vi "Test Copy All Funnels.vi"(8 "error in (no error)":errorcluster) -> (0 "error out":errorcluster)   [LabVIEW 2019]
uses:
  Setting Database/Setting Database.lvclass
  C:/Program Files (x86)/National Instruments/LabVIEW 2019/vi.lib/JKI/JKI SMO/SMO/SMO.lvclass
  Setting Database/Typedefs/PrivateEvents--Setting Database.CopyActiveFunnelToAll.ctl
  ObjectSettings/ObjectSettings.lvclass/ObjectSettings.ctl
  ObjectSettings/Accessors/Read Enabled.vi
  ObjectSettings/Accessors/Write Enabled.vi
  Funnel Settings/Funnel Settings.lvclass
  C:/Users/Albro/Documents/GitHub/AFM-Lithography/lvsrc/Classes/Settings/ObjectSettings/ObjectSettings.lvclass
  <vilib>/addons/_JKI Toolkits/Caraya/classes/Assert/Assert Equal Value_Variant.vi
  <vilib>/addons/_JKI Toolkits/Caraya/classes/Assert/Assert Not Error.vi
  <vilib>/addons/_JKI Toolkits/Caraya/classes/Test/Test.lvclass
  <vilib>/addons/_JKI Toolkits/Caraya/classes/Assert/Assert.lvclass
  <vilib>/JKI/JKI SMO/SMO/SMO.lvclass
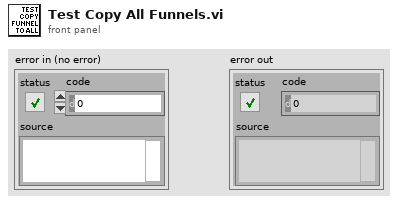
[diagram p1: front panel]
types:
  T1 = typedef "Setting Database.lvclass/PrivateEvents--Setting Database.CopyActiveFunnelToAll.ctl" = bool
  T2 = typedef "Setting Database.lvclass/PublicEvents--Cluster.ctl" = cluster{"NewActivePath":refnum<user-event>, "PathsUpdated":refnum<user-event>, "RectanglesUpdated":refnum<user-event>, "NewActiveRectangle":refnum<user-event>, "NewActiveFunnel":refnum<user-event>, "FunnelsUpdated":refnum<user-event>, "NewActiveDot":refnum<user-event>, "DotsUpdated":refnum<user-event>}
  T3 = typedef "Setting Database.lvclass/PrivateEvents--Setting Database.Refresh.ctl" = cluster{"Paths":string[], "Rectangles":string[], "Funnels":string[], "Dots":string[]}
  T4 = typedef "Setting Database.lvclass/PublicEvents--Setting Database.NewActiveFunnel.ctl" = refnum<class "Funnel Settings.lvclass">
  T5 = typedef "Setting Database.lvclass/PublicEvents--Setting Database.FunnelsUpdated.ctl" = refnum<class "Funnel Settings.lvclass">[]
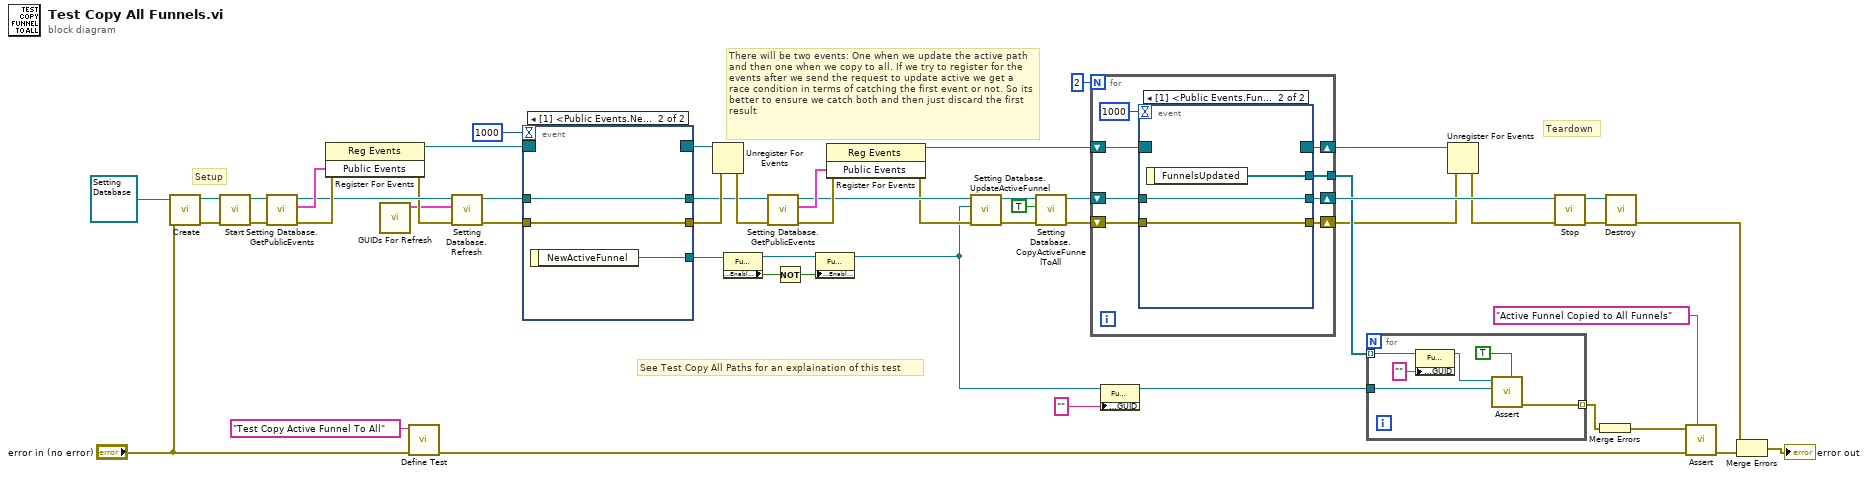
[diagram p0: block diagram]
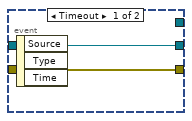
[diagram p2: hidden frame]
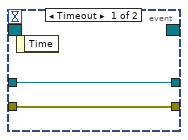
[diagram p3: hidden frame]
diagram:
  # "See Test Copy All Paths for an explaination of this test"
  # "There will be two events: One when we update the active path and then one when we copy to all. If we try to register for the events after we send the request to update active we get a race condition in terms of catching the first event or not. So its better to ensure we catch both and then just discard the first result"
  # "Teardown"
  # "Setup"
  n1 = call <vilib>:"Create.vi"("error in (no error)"="error in (no error)", "SMO"=refnum<class "Setting Database.lvclass"> refnum ("Setting Database.lvclass")) -> ("error out"=w49:errorcluster, "SMO out"=w40:refnum<class "Setting Database.lvclass">)  [unwired: 7 in, 1 out]
  n2 = call <vilib>:"Start.vi"("error in (no error)"=w49, "SMO"=w40) -> ("error out"=w48:errorcluster, "SMO out"=w39:refnum<class "Setting Database.lvclass">)  [unwired: 8 in]
  n3 = call "Setting Database.GetPublicEvents.vi"("error in (no error)"=w48, "Setting Database"=w39) -> ("error out"=w45:errorcluster, "Public Events"=w34:T2, "Setting Database out"=w32:refnum<class "Setting Database.lvclass">)  [unwired: 7 in]
  n4 = register-events(error in=w45, w34) -> (reference out=w35:refnum<event-registration>, error out=w31:errorcluster)  [unwired: 1 in]
  n5 = call "GUIDs For Refresh.vi"() -> ("Initialize"=w4:T3)  [unwired: 10 in, 1 out]
  n6 = call <vilib>:"Define Test.vi"("error in (no error)"="error in (no error)", "Label (VI Title)"="Test Copy Active Funnel To All") -> ("error out"=w51:errorcluster)  [unwired: 8 in, 1 out]
  n7 = call "Setting Database.Refresh.vi"("error in (no error)"=w31, "Initialize"=w4, "Setting Database"=w32) -> ("error out"=w30:errorcluster, "Setting Database out"=w29:refnum<class "Setting Database.lvclass">)  [unwired: 7 in]
  n8 = event shown="[1] <Public Events.NewActiveFunnel>: User Event" {
    selector: w35 -> [_ _]
    dyn-events: [_ _] -> w37
    timeout: 1000 -> [_ _]
    tunnel: [w54 w57] -> w46
    tunnel: w30 -> [w54 w57]
    tunnel: w29 -> [w53 w56]
    tunnel: [w53 w56] -> w17
    tunnel: [_ w55] -> w28
    event Timeout {
      n9 = event-data() -> ()  [unwired: 1 in, 1 out]
    }
    event User Event {
      n10 = event-data() -> ("NewActiveFunnel"=w55:T4)  [unwired: 1 in]
    }
  }
  n11 = Unregister For Events(event registration refnum=w37, error in=w46) -> (error out=w18:errorcluster)
  n12 = property on="Property Node" class="Funnel Settings.lvclass"(reference=w28) -> (reference out=w27:T4, "Accessors:Enabled"=w26:bool)  [unwired: 1 in, 1 out]
  n13 = call "Setting Database.GetPublicEvents.vi"("error in (no error)"=w18, "Setting Database"=w17) -> ("error out"=w16:errorcluster, "Public Events"=w24:T2, "Setting Database out"=w11:refnum<class "Setting Database.lvclass">)  [unwired: 7 in]
  n14 = Not(x=w26) -> (.not. x?=w25:bool)
  n15 = property on="Property Node" class="Funnel Settings.lvclass"(reference=w27, "Accessors:Enabled"=w25) -> (reference out=w2:T4)  [unwired: 1 in, 1 out]
  n16 = register-events(error in=w16, w24) -> (reference out=w22:refnum<event-registration>, error out=w10:errorcluster)  [unwired: 1 in]
  n17 = call "Setting Database.UpdateActiveFunnel.vi"("error in (no error)"=w10, "UpdateActiveFunnel"=w2, "Setting Database"=w11) -> ("error out"=w7:errorcluster, "Setting Database"=w9:refnum<class "Setting Database.lvclass">)  [unwired: 7 in]
  n18 = call "Setting Database.CopyActiveFunnelToAll.vi"("error in (no error)"=w7, "CopyActiveFunnelToAll"=T1 TRUE, "Setting Database"=w9) -> ("error out"=w6:errorcluster, "Setting Database out"=w8:refnum<class "Setting Database.lvclass">)  [unwired: 7 in]
  n19 = for {
    N: 2 -> [_]
    tunnel: [w60] -> w21
    shift-right: [w64] -> w23
    shift-left: w8 -> [w65]
    shift-right: [w63] -> w13
    shift-left: w6 -> [w62]
    shift-right: [w59] -> w14
    shift-left: w22 -> [w61]
    n20 = event shown="[1] <Public Events.FunnelsUpdated>: User Event" {
      selector: w61 -> [_ _]
      dyn-events: [_ _] -> w59
      timeout: 1000 -> [_ _]
      tunnel: w65 -> [w67 w70]
      tunnel: [w67 w70] -> w64
      tunnel: [w66 w69] -> w63
      tunnel: w62 -> [w66 w69]
      tunnel: [_ w68] -> w60
      event Timeout {
        n21 = event-data() -> ()  [unwired: 1 in, 3 out]
      }
      event User Event {
        n22 = event-data() -> ("FunnelsUpdated"=w68:T5)  [unwired: 1 in]
      }
    }
  }
  n23 = property on="Property Node" class="Funnel Settings.lvclass"(reference=w2, "Accessors:GUID"="" ("GUID")) -> (reference out=w1:T4)  [unwired: 1 in, 1 out]
  n24 = for {
    tunnel: w21 -> [w72] mode=indexing
    tunnel: w1 -> [w76]
    tunnel: [w75] -> w20 mode=indexing
    n25 = property on="Property Node" class="Funnel Settings.lvclass"(reference=w72, "Accessors:GUID"="" ("GUID")) -> (reference out=w73:refnum<class "Funnel Settings.lvclass">)  [unwired: 1 in, 1 out]
    n26 = call-poly <vilib>:"Assert.vi"("Assert Only? (F)"=TRUE, "Actual"=w76, "Expected"=w73) -> ("error out"=w75:errorcluster)  [unwired: 7 in, 1 out]
  }
  n27 = Unregister For Events(event registration refnum=w14, error in=w13) -> (error out=w12:errorcluster)
  n28 = call <vilib>:"Stop.vi"("error in (no error)"=w12, "SMO"=w23) -> ("error out"=w47:errorcluster, "SMO out"=w38:refnum<class "Setting Database.lvclass">)  [unwired: 8 in]
  n29 = Merge Errors(w20) -> (w19:errorcluster)
  n30 = call <vilib>:"Destroy.vi"("error in (no error)"=w47, "SMO"=w38) -> ("error out"=w44:errorcluster)  [unwired: 9 in]
  n31 = call-poly <vilib>:"Assert.vi"("Label"="Active Funnel Copied to All Funnels" ("Label (VI Title)"), "error in (no error)"=w51, "Not Error?"=w19) -> ("error out"=w52:errorcluster)  [unwired: 7 in, 1 out]
  n32 = Merge Errors(w44, w52) -> (→"error out":errorcluster)
